vi "Cleanup.vi"(8 "error in (no error)":errorcluster, 11 "Ambient Light Bricklet in":refnum<class "IO-4 Bricklet.lvclass">) -> (0 "error out":errorcluster)   [LabVIEW 2011, in "Tinkerforge.lvlib" / "IO-4 Bricklet.lvclass"]
doc: "This VI is the child implementation of \"Cleanup.vi\" and releases all synchronization objects of this child object."
uses:
  IO-4 Bricklet.lvclass
  IO-4 Bricklet.lvclass/IO-4 Bricklet.ctl
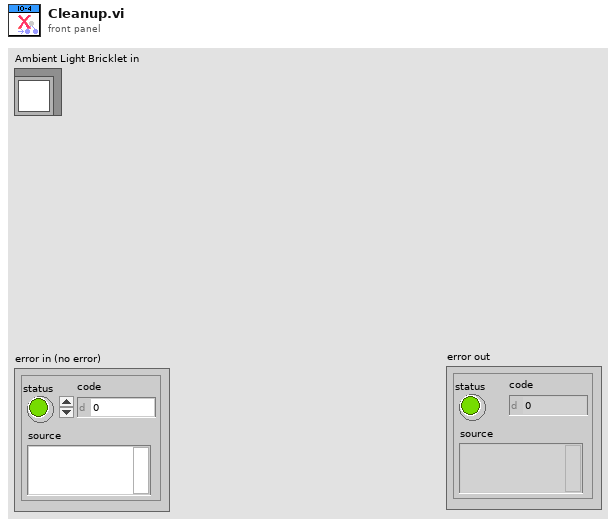
[diagram p1: front panel]
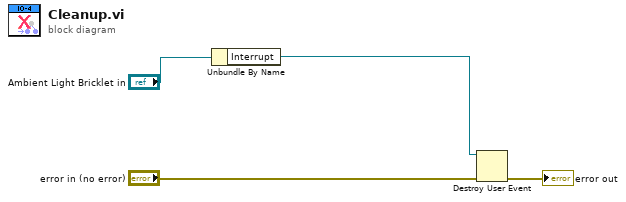
[diagram p0: block diagram]
diagram:
  n1 = Unbundle By Name("Ambient Light Bricklet in") -> ("Interrupt"=w2:refnum<user-event>)
  n2 = Destroy User Event(user event=w2, error in="error in (no error)") -> (error out=→"error out":errorcluster)
